vi "GetPrivateQueueConfig.vi"(8 "error in (no error)":errorcluster, 11 "DAQmx":refnum<class "DAQmx.lvclass">) -> (0 "error out":errorcluster, 3 "DAQmx out":refnum<class "DAQmx.lvclass">)   [LabVIEW 2019, in "DAQmx.lvclass"]
uses:
  DAQmx.lvclass
  DAQmx.lvclass/DAQmx.ctl
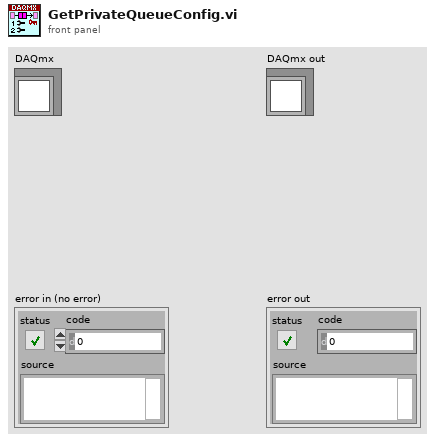
[diagram p1: front panel]
types:
  T1 = typedef "DAQmx.lvclass/DAQ.Config.Timing--Cluster.ctl" = cluster{"Sampling":T2, "Fs_Out":dbl}
  T2 = typedef "DAQmx.lvclass/DAQ.Config.Timing.Sampling--Cluster.ctl" = cluster{"Fs":dbl, "#s":i32}
  T3 = typedef "DAQmx.lvclass/DAQ.Config.AO--Cluster--Array.ctl" = T4[]
  T4 = typedef "DAQmx.lvclass/DAQ.Config.AO--Cluster.ctl" = cluster{"Channels":tag, "Range":T5, "output terminal configuration":i32, "Type":T6}
  T5 = typedef "DAQmx.lvclass/DAQ.Config.AO.Range--enum.ctl" = enum16{"±0.1", "±1.0", "±3.5", "±10.0", ""}
  T6 = typedef "DAQmx.lvclass/DAQ.Config.Device Type--enum.ctl" = enum16{"None", "USB-4431", "PXI-446x"}
  T7 = typedef "DAQmx.lvclass/DAQ.Config.AI--Cluster--Array.ctl" = T8[]
  T8 = typedef "DAQmx.lvclass/DAQ.Config.AI--Cluster.ctl" = cluster{"Channels":tag, "Coupling":T9, "Range":T10, "input terminal configuration":i32, "Type":T6}
  T9 = typedef "DAQmx.lvclass/DAQ.Config.AI.Coupling--enum.ctl" = u16
  T10 = typedef "DAQmx.lvclass/DAQ.Config.AI.Range--enum.ctl" = enum16{"±0.316", "±1.00", "±3.16", "±10.0", "±31.6", "±42.4", ""}
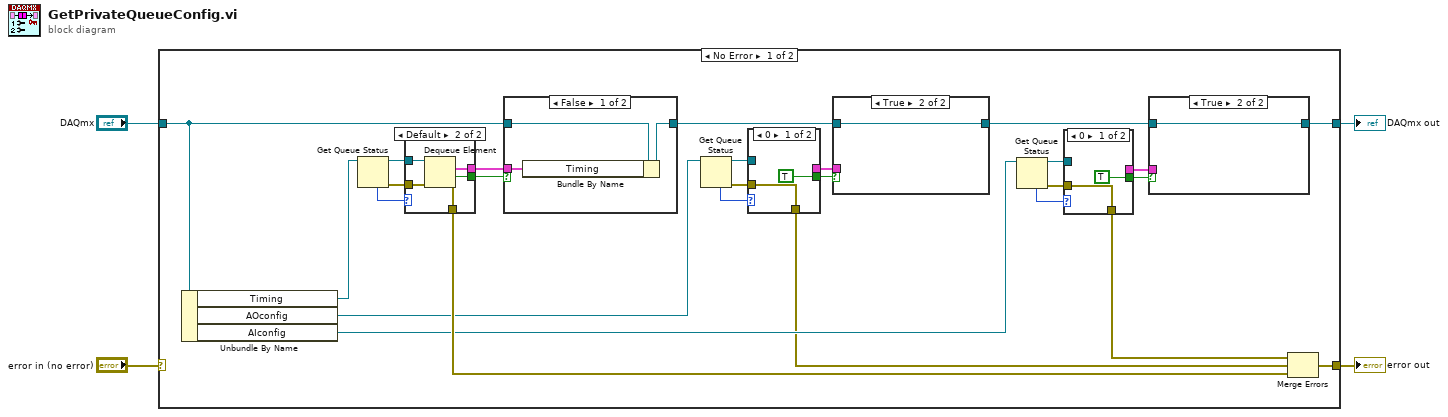
[diagram p0: block diagram]
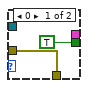
[diagram p2: hidden frame]
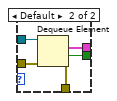
[diagram p3: hidden frame]
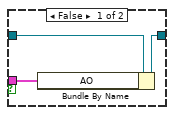
[diagram p5: hidden frame]
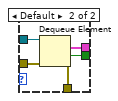
[diagram p6: hidden frame]
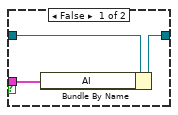
[diagram p7: hidden frame]
diagram:
  n1 = case shown="No Error" "error in (no error)" {
    selector: "error in (no error)" -> [_ w65]
    tunnel: [w30 w64] -> w4
    tunnel: [w25 w65] -> w2
    tunnel: "DAQmx" -> [w5 w64]
    frame No Error {
      n2 = Unbundle By Name(w5) -> ("Timing"=w23:refnum<queue>, "AOconfig"=w12:refnum<queue>, "AIconfig"=w13:refnum<queue>)
      n3 = Get Queue Status(queue=w23) -> (queue out=w22:refnum<queue>, error out=w20:errorcluster, # elements in queue=w21:i32)  [unwired: 2 in, 5 out]
      n4 = case shown="Default" w21 {
        tunnel: [_ w37] -> w29
        tunnel: [TRUE ("timed out?") w36] -> w28
        tunnel: [w31 w35] -> w24
        tunnel: w22 -> [_ w34]
        tunnel: w20 -> [w31 w33]
        frame 0 {
        }
        frame Default {
          n5 = Dequeue Element(queue=w34, error in (no error)=w33) -> (element=w37:T1, timed out?=w36:bool, error out=w35:errorcluster)  [unwired: 1 in, 1 out]
        }
      }
      n6 = case shown="False" w28 {
        tunnel: w5 -> [w47 w48]
        tunnel: [w46 w48] -> w27
        tunnel: w29 -> [w45 _]
        frame False {
          n7 = Bundle By Name(cluster=w47, "Timing"=w45) -> (w46:refnum<class "DAQmx.lvclass">)
        }
        frame True {
        }
      }
      n8 = Get Queue Status(queue=w12) -> (queue out=w19:refnum<queue>, error out=w17:errorcluster, # elements in queue=w18:i32)  [unwired: 2 in, 5 out]
      n9 = case shown="0" w18 {
        tunnel: [_ w44] -> w9
        tunnel: [TRUE ("timed out?") w43] -> w8
        tunnel: [w38 w42] -> w11
        tunnel: w19 -> [_ w41]
        tunnel: w17 -> [w38 w40]
        frame 0 {
        }
        frame Default {
          n10 = Dequeue Element(queue=w41, error in (no error)=w40) -> (element=w44:T3, timed out?=w43:bool, error out=w42:errorcluster)  [unwired: 1 in, 1 out]
        }
      }
      n11 = case shown="True" w8 {
        tunnel: w27 -> [w51 w52]
        tunnel: [w50 w52] -> w26
        tunnel: w9 -> [w49 _]
        frame False {
          n12 = Bundle By Name(cluster=w51, "AO"=w49) -> (w50:refnum<class "DAQmx.lvclass">)
        }
        frame True {
        }
      }
      n13 = Get Queue Status(queue=w13) -> (queue out=w16:refnum<queue>, error out=w14:errorcluster, # elements in queue=w15:i32)  [unwired: 2 in, 5 out]
      n14 = case shown="0" w15 {
        tunnel: [_ w59] -> w6
        tunnel: [TRUE ("timed out?") w58] -> w7
        tunnel: [w53 w57] -> w10
        tunnel: w16 -> [_ w56]
        tunnel: w14 -> [w53 w55]
        frame 0 {
        }
        frame Default {
          n15 = Dequeue Element(queue=w56, error in (no error)=w55) -> (element=w59:T7, timed out?=w58:bool, error out=w57:errorcluster)  [unwired: 1 in, 1 out]
        }
      }
      n16 = case shown="True" w7 {
        tunnel: w26 -> [w62 w63]
        tunnel: [w61 w63] -> w30
        tunnel: w6 -> [w60 _]
        frame False {
          n17 = Bundle By Name(cluster=w62, "AI"=w60) -> (w61:refnum<class "DAQmx.lvclass">)
        }
        frame True {
        }
      }
      n18 = Merge Errors(w10, w11, w24) -> (w25:errorcluster)
    }
    frame Error {
    }
  }
  "error out" <- w2
  "DAQmx out" <- w4
